vi "Write Bacta [l].vi"(8 "error in (no error)":errorcluster, 10 "Bacta [l]":u8 max=10, 11 "MedicalDroid in":refnum<class "MedicalDroid.lvclass">) -> (0 "error out":errorcluster, 3 "MedicalDroid out":refnum<class "MedicalDroid.lvclass">)   [LabVIEW 2021, in "MedicalDroid.lvclass"]
uses:
  MedicalDroid.lvclass
  MedicalDroid.lvclass/MedicalDroid.ctl
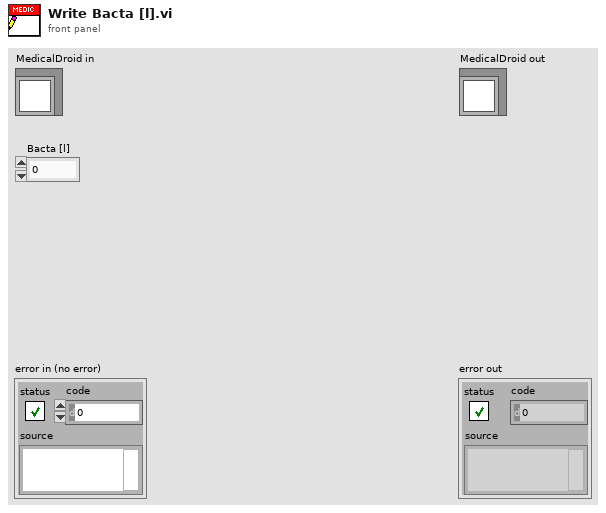
[diagram p1: front panel]
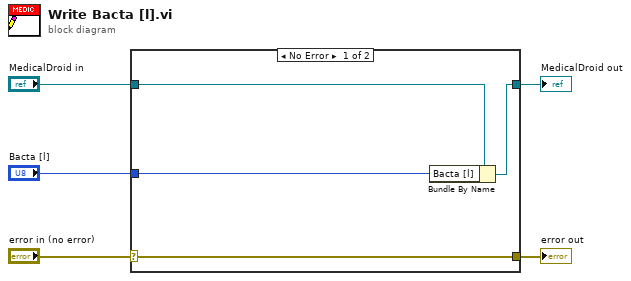
[diagram p0: block diagram]
diagram:
  n1 = case shown="No Error" "error in (no error)" {
    selector: "error in (no error)" -> [w9 w10]
    tunnel: [w9 w10] -> w4
    tunnel: [w7 w11] -> w2
    tunnel: "MedicalDroid in" -> [w8 w11]
    tunnel: "Bacta [l]" -> [w6 _]
    frame No Error {
      n2 = Bundle By Name(cluster=w8, "Bacta [l]"=w6) -> (w7:refnum<class "MedicalDroid.lvclass">)
    }
    frame Error {
    }
  }
  "error out" <- w4
  "MedicalDroid out" <- w2
